vi "arreglos.vi"() -> ()   [LabVIEW 2020]
uses:
  fff0bf57-45df-46f0-a67c-803726d23d77.vi
  158622c4-690d-470d-afd1-f132748040d2.vi
panel:
  out "array out 2":dbl[](array[numeric])
  out "array out":dbl[](array[numeric])
  out "index of element":i32
  out "output array 3":dbl[][](array[numeric])
  out "min index(es)":i32
  out "max index(es)":i32
  out "min value":dbl
  out "max value":dbl
  out "subarray":dbl[](array[numeric])
  out "appended array":dbl[](array[numeric])
  in  "Numeric 5":dbl
  in  "Numeric 4":dbl
  in  "Numeric 3":dbl
  in  "Numeric 2":dbl
  in  "Numeric":dbl
  out "initialized array 2":bool[](array[boolean])
  out "initialized array":dbl[](array[numeric])
  out "deleted portion":dbl[](array[numeric])
  out "array w/ subset deleted":dbl[](array[numeric])
  out "output array 2":dbl[](array[numeric])
  in  "tacometro":dbl(knob) scale=0.0..10.0
  in  "velocidad":dbl(knob) scale=0.0..10.0
  out "size(s)":i32
  in  "Array":dbl[](array[slide]) scale=0.0..10.0
  out "element 5":string
  out "output array":bool[](array[boolean])
  out "element 4":dbl
  out "element 3":dbl
  out "element 2":dbl
  out "element":dbl
  in  "arreglo string":string[](array[string])
  in  "arreglo bool":bool[](array[boolean])
  in  "arreglo double":dbl[](array[slide]) scale=0.0..100.0
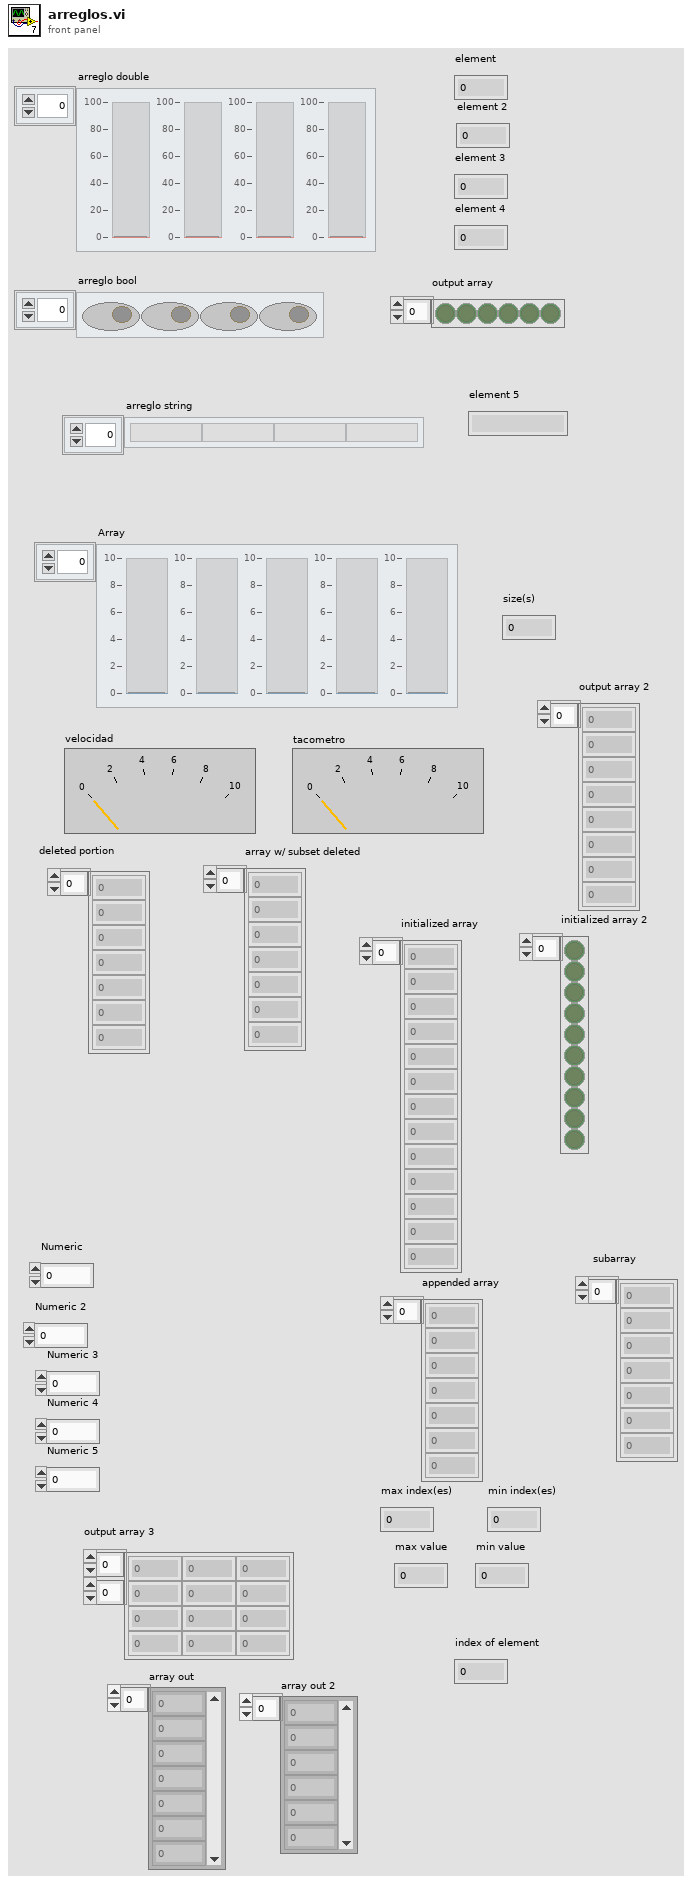
[diagram p1: front panel]
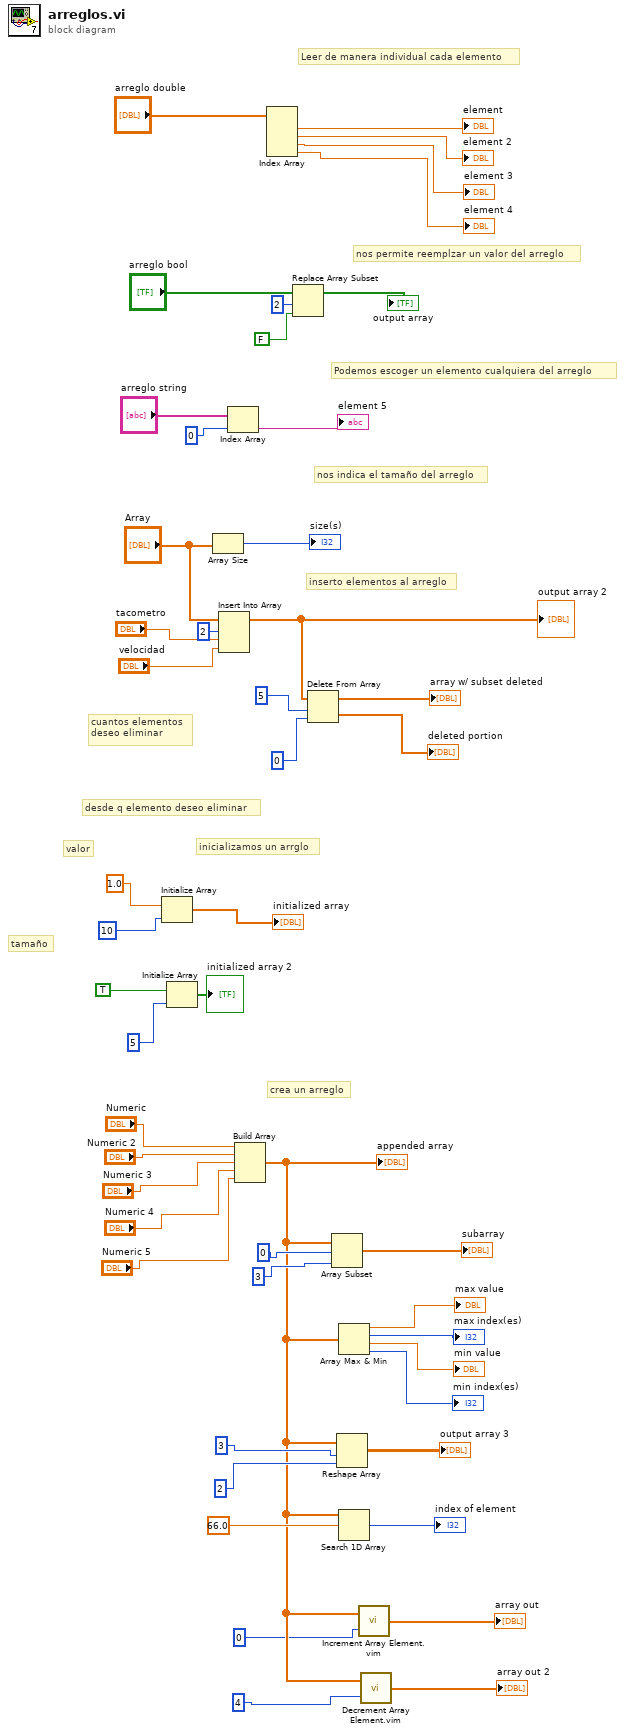
[diagram p0: block diagram]
diagram:
  # "crea un arreglo"
  # "tamaño"
  # "valor"
  # "inicializamos un arrglo"
  # "desde q elemento deseo eliminar"
  # "cuantos elementos\ndeseo eliminar"
  # "inserto elementos al arreglo"
  # "nos indica el tamaño del arreglo"
  # "Podemos escoger un elemento cualquiera del arreglo"
  # "nos permite reemplzar un valor del arreglo"
  # "Leer de manera individual cada elemento"
  n1 = Initialize Array(1.0, 10) -> (→"initialized array":dbl[])
  n2 = Initialize Array(TRUE, 5 ("dimension size")) -> (→"initialized array 2":bool[])
  n3 = Array Size(array="Array") -> (size(s)=→"size(s)":i32)
  n4 = Insert Into Array(array="Array", index=2, new element #1="tacometro", new element #2="velocidad") -> (w33:dbl[])
  "output array 2" <- w33
  n5 = Index Array(array="arreglo string", index=0) -> (element=→"element 5":string)
  n6 = Build Array("Numeric", "Numeric 2", "Numeric 3", "Numeric 4", "Numeric 5") -> (w5:dbl[])
  "appended array" <- w5
  n7 = Index Array(array="arreglo double") -> (element #1=→"element":dbl, element #2=→"element 2":dbl, element #3=→"element 3":dbl, element #4=→"element 4":dbl)  [unwired: 4 in]
  n8 = Replace Array Subset(array="arreglo bool", new element=FALSE, index=2) -> (→"output array":bool[])
  n9 = Delete From Array(array=w33, length=5, index=0) -> (deleted portion=→"deleted portion":dbl[], array with subset deleted=→"array w/ subset deleted":dbl[])
  n10 = Array Subset(array=w5, index=0 ("dimension size"), length=3 ("dimension size")) -> (→"subarray":dbl[])
  n11 = Reshape Array(w5, 3 ("dimension size"), 2 ("dimension size")) -> (→"output array 3":dbl[][])
  n12 = Array Max & Min(array=w5) -> (max value=→"max value":dbl, max index (indices)=→"max index(es)":i32, min value=→"min value":dbl, min index (indices)=→"min index(es)":i32)
  n13 = Search 1D Array(1D array=w5, element=66.0) -> (index of element=→"index of element":i32)  [unwired: 1 in]
  n14 = call "Increment Array Element.vim"("index"=0 ("dimension size"), "array in"=w5) -> ("array out"=→"array out":dbl[])
  n15 = call "Decrement Array Element.vim"("index"=4 ("dimension size"), "array in"=w5) -> ("array out"=→"array out 2":dbl[])
